vi "CanChannelReadMsg.vi"(0 "CAN Channel Handle in":u32 format="%x", 1 "Milliseconds":u32=4294967295 format="%x", 2 "error in":errorcluster {"code" format="%.0x"}) -> (3 "CAN Channel Handle out":u32, 4 "Is Valid Message":bool, 5 "CAN message":T1 {"DLC" max=8; "Data"."[4]" format="%02x"; "Data"."[7]" format="%02x"; "Data"."[6]" format="%02x"; "Data"."[5]" format="%02x"; "Data"."[3]" format="%02x"; "Data"."[2]" format="%02x"; "Data"."[1]" format="%02x"; "Data"."[0]" format="%02x"; "Timestamp" format="%08x"; "Arbitration ID" format="%08x"}, 6 "error out":errorcluster {"code" format="%.0x"})   [LabVIEW 2012]
doc: "Reads the next CAN message from the receive FIFO of the channel."
uses:
  vcilva.dll
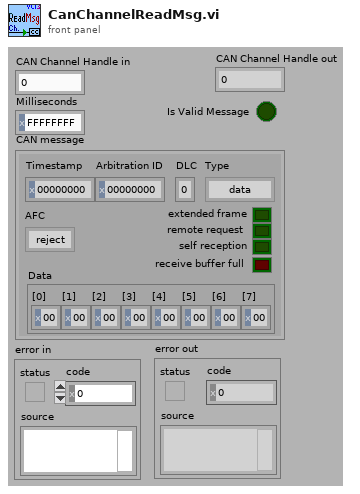
[diagram p1: front panel]
types:
  T1 = cluster{"Timestamp":u32, "Arbitration ID":u32, "DLC":u8, "Type":enum8{"data", "info", "error", "status", "wakeup", "timer ovr", "timer reset"}, "AFC":enum8{"reject", "always", "filter 1", "filter 2"}, "extended frame":bool, "remote request":bool, "self reception":bool, "receive buffer full":bool, "Data":cluster{"[0]":u8, "[1]":u8, "[2]":u8, "[3]":u8, "[4]":u8, "[5]":u8, "[6]":u8, "[7]":u8}}
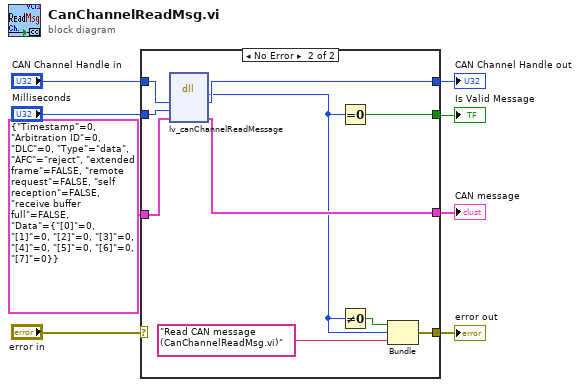
[diagram p0: block diagram]
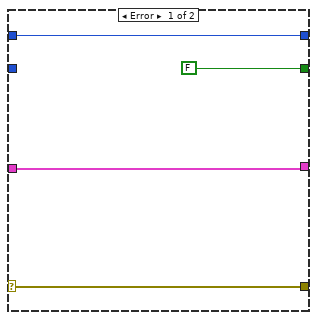
[diagram p2: hidden frame]
diagram:
  n1 = case shown="No Error" "error in" {
    selector: "error in" -> [w12 _]
    tunnel: [w12 w22] -> w8
    tunnel: "CAN Channel Handle in" -> [w11 w20]
    tunnel: [w11 w17] -> w6
    tunnel: [w9 w18] -> w1
    tunnel: "Milliseconds" -> [_ w19]
    tunnel: [FALSE w15] -> w3
    tunnel: T1 {"Timestamp"=0, "Arbitration ID"=0, "DLC"=0, "Type"=enum."data", "AFC"=enum."reject", "extended frame"=FALSE, "remote request"=FALSE, "self reception"=FALSE, "receive buffer full"=FALSE, "Data"={"[0]"=0, "[1]"=0, "[2]"=0, "[3]"=0, "[4]"=0, "[5]"=0, "[6]"=0, "[7]"=0}} ("CAN message") -> [w9 w13]
    frame Error {
    }
    frame No Error {
      n2 = dll-call lib="vcilva.dll" fn="lv_canChannelReadMessage"("hCanChn"=w20, "dwMilliseconds"=w19, "CAN message"=w13) -> (w14:i32, "hCanChn"=w17:u32, "CAN message"=w18:T1)  [unwired: 4 in, 2 out]
      n3 = Equal To 0?(x=w14) -> (x = 0?=w15:bool)
      n4 = Not Equal To 0?(x=w14) -> (x != 0?=w16:bool)
      n5 = Bundle(w16, w14, "Read CAN message (CanChannelReadMsg.vi)") -> (w22:errorcluster)  [unwired: 1 in]
    }
  }
  "error out" <- w8
  "CAN Channel Handle out" <- w6
  "Is Valid Message" <- w3
  "CAN message" <- w1
